vi "Read From Spreadsheet_LV2012_NI Verified.vi"(7 "My File has Row Headers":bool=TRUE, 9 "Data Precision":i16=3, 11 "Spreadsheet path (.csv)":path) -> (2 "Data Display":i64[][](array[numeric]), 3 "Spread Sheet Display":string[][](array[string]))   [LabVIEW 2017]
doc: "This example shows how you can use the Read from Spreadsheet VI to pull data from a spreadsheet."
uses:
  <vilib>/Utility/file.llb/Read From Spreadsheet File (string).vi
  <vilib>/Utility/file.llb/Read From Spreadsheet File (I64).vi
panel:
  # "Overview: This example shows how you can use the Read from Spreadsheet VI to pull data from a spreadsheet.\nRequirements: LabVIEW 2012( or compatible)\nInstructions:\n1. Choose the path of the CSV File: Browse to the folder where this VI is stored and choose Data.csv\n2. Choose the Data Precision you would like to display\n3. Click on My File has Row Headers if the file has headers\n4. Run the VI"
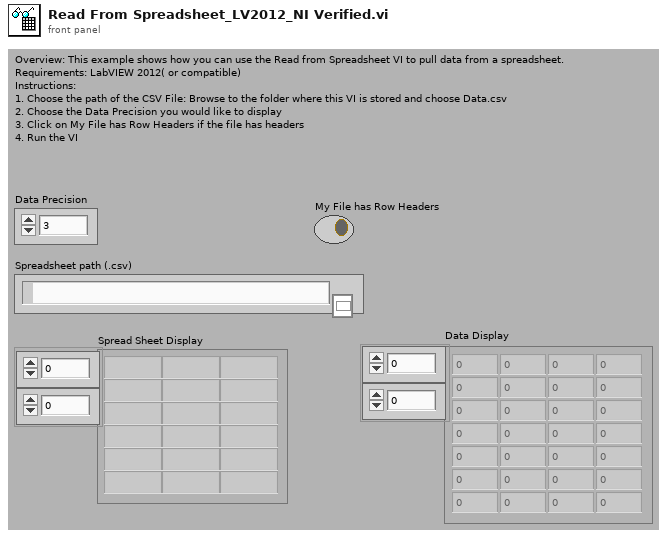
[diagram p1: front panel]
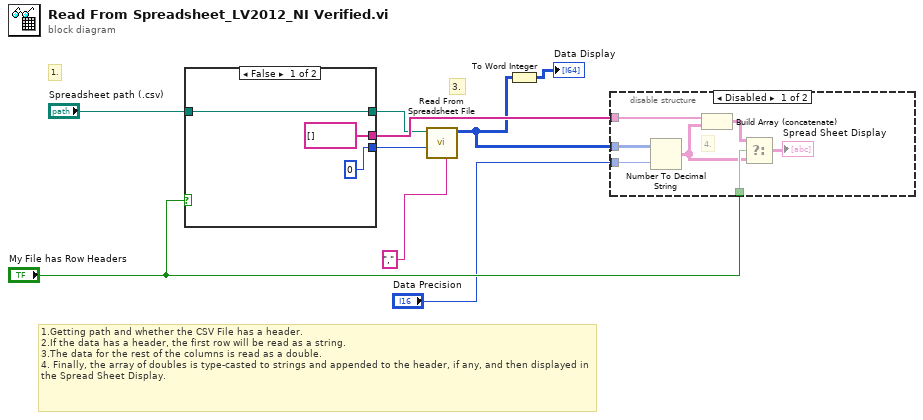
[diagram p0: block diagram]
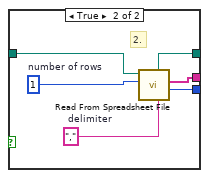
[diagram p3: hidden frame]
diagram:
  # "1.Getting path and whether the CSV File has a header.\n2.If the data has a header, the first row will be read as a string.\n3.The data for the rest of the columns is read as a double.\n4. Finally, the array of doubles is type-casted to strings and appended to the header, if any, and then displayed in the Spread Sheet Display."
  # "3."
  # "1."
  n1 = case shown="False" "My File has Row Headers" {
    tunnel: "Spreadsheet path (.csv)" -> [w10 w18]
    tunnel: [string[] [] ("first row") w16] -> w7
    tunnel: [0 ("mark after read (chars.)") w15] -> w4
    tunnel: [w10 w13] -> w6
    frame False {
    }
    frame True {
      w14 = 1  # number of rows
      w17 = ","  # delimiter
      # "2."
      n2 = call-poly <vilib>:"Read From Spreadsheet File.vi"("delimiter (\\t)"=w17, "number of rows (all:-1)"=w14, "file path (dialog if empty)"=w18) -> ("mark after read (chars.)"=w15:i32, "first row"=w16:string[], "new file path (Not A Path if cancelled)"=w13:path)  [unwired: 4 in, 2 out]
    }
  }
  n3 = call-poly <vilib>:"Read From Spreadsheet File.vi"("delimiter (\\t)"="," ("delimiter (\\t)"), "start of read offset (chars.:0)"=w4, "file path (dialog if empty)"=w6) -> ("all rows"=w2:i64[][])  [unwired: 4 in, 4 out]
  n4 = To Word Integer(number=w2) -> (16bit integer=→"Data Display":i16[][])
  n5 = disable-structure shown="Disabled" {
    disable-tunnel: w7 -> [w25 _]
    disable-tunnel: "My File has Row Headers" -> [w23 _]
    disable-tunnel: w2 -> [w20 _]
    disable-tunnel: "Data Precision" -> [w19 _]
    frame Disabled {
      # "4."
      n6 = Number To Decimal String(number=w20, width (-)=w19) -> (decimal integer string=w21:string[][])
      n7 = Build Array (concatenate)(w25, w21) -> (w24:string[][])
      n8 = Select(t=w24, s=w23, f=w21) -> (s? t:f=→"Spread Sheet Display":string[][])
    }
    frame Enabled {
    }
  }
